vi "ini-to-toml.vi"(8 "error in":errorcluster, 11 "ini file":path) -> (0 "error out":errorcluster, 2 "toml file":path)   [LabVIEW 2020, in "configuration-data.lvclass"]
uses:
  configuration-data.lvclass
  configuration-data.lvclass/configuration-data.ctl
  45fe5cc2-d305-4dac-bcbd-01e3c5dbc327.vi
  configuration.get.vi
  configuration.set.vi
  <vilib>/Utility/config.llb/Open Config Data.vi
  <vilib>/Utility/config.llb/Get Section Names.vi
  <vilib>/Utility/config.llb/Get Key Names.vi
  <vilib>/Utility/config.llb/Read Key.vi
  <vilib>/Utility/config.llb/Read Key (String).vi
  datatype_conversion.vi
  <vilib>/Utility/config.llb/Close Config Data.vi
  <userlib>/_OpenG.lib/file/file.llb/Convert File Extension (Path)__ogtk.vi
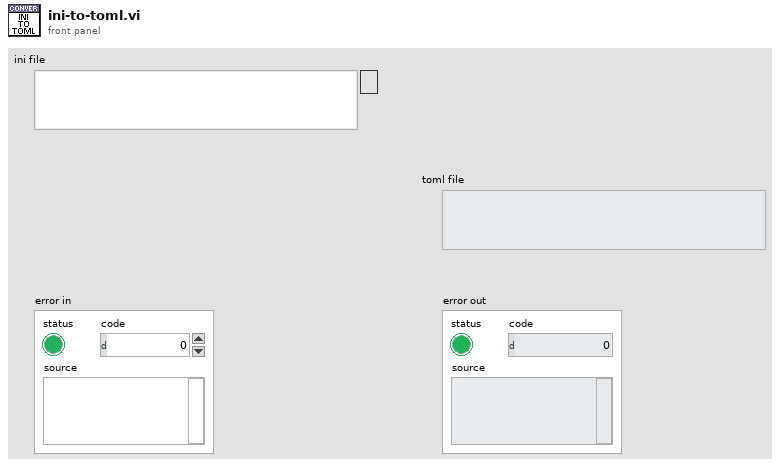
[diagram p1: front panel]
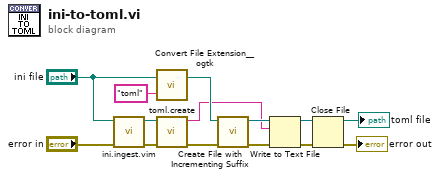
[diagram p0: block diagram]
diagram:
  n1 = call "ini.ingest.vim"("error in"="error in", "config string or path"="ini file") -> ("error out"=w13:errorcluster, "configuration-data"=w14:refnum<class "configuration-data.lvclass">)  [unwired: 8 in]
  n2 = call-poly <userlib>:"Convert File Extension__ogtk.vi"("new ending (none)"="toml", "file name"="ini file") -> ("new filename"=w9:path)  [unwired: 1 out]
  n3 = call "toml.create.vi"("error in"=w13, "configuration-data"=w14) -> ("error out"=w8:errorcluster, "toml"=w5:string)  [unwired: 8 in]
  n4 = call <vilib>:"Create File with Incrementing Suffix.vi"("error in (no error)"=w8, "file path"=w9) -> ("error out"=w6:errorcluster, "refnum out"=w7:refnum<file>)  [unwired: 7 in, 1 out]
  n5 = Write to Text File(file (use dialog)=w7, text=w5, error in=w6) -> (refnum out=w4:refnum<file>, error out=w3:errorcluster)  [unwired: 1 in, 1 out]
  n6 = Close File(refnum=w4, error in=w3) -> (path=→"toml file":path, error out=→"error out":errorcluster)
